vi "CreateS19Data.vi"(0 "SoftwareFilesPath [C:\\PRUEF]":string="C:\\PRUEF\\Programming\\001.001.001pre", 1 "Address [hex - 4bit]":u32=4198400 format="%08x", 2 "DataType":u16(ring) items=["ASCI", "FourByteCalData", "Hex"], 3 "Data [ASCII]":string="Empty", 4 "calData":u32 format="%.0x", 5 "Data":u8[](array[numeric]) format="%.0x", 6 "append?":bool) -> (19 "error out":errorcluster)   [LabVIEW 2012]
panel:
  out "spreadsheet string":string="S30B004010004FF003007047AB"
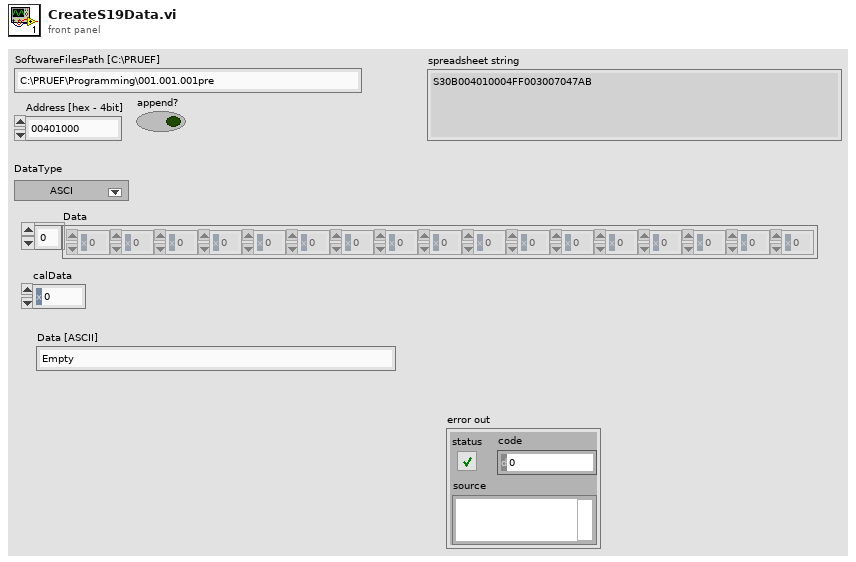
[diagram p1: front panel]
types:
  T1 = enum16{"open", "replace", "create", "open or create", "replace or create", "replace or create with confirmation"}
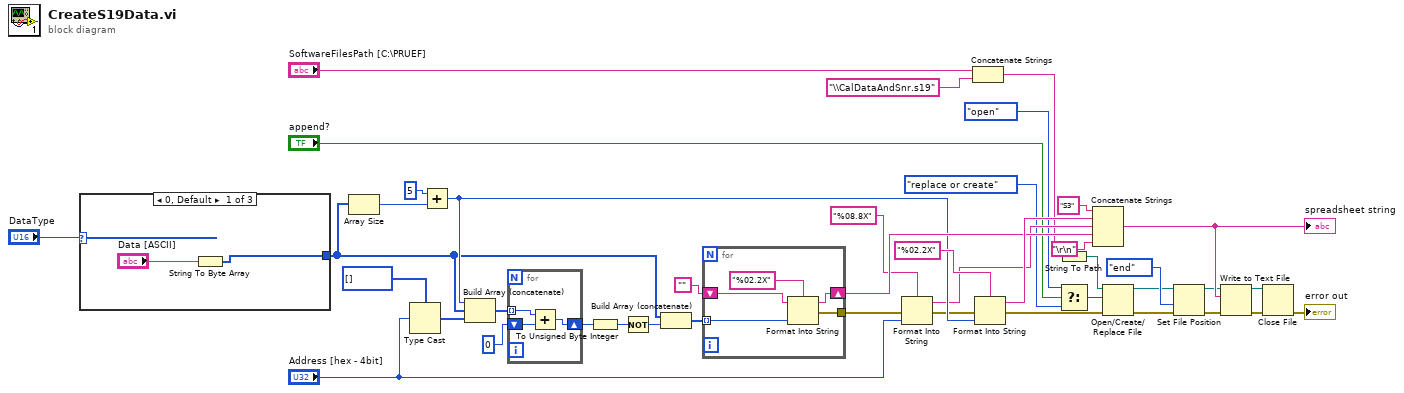
[diagram p0: block diagram]
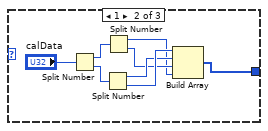
[diagram p2: hidden frame]
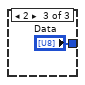
[diagram p3: hidden frame]
diagram:
  n1 = case shown="0, Default" "DataType" {
    tunnel: [w43 w45 "Data"] -> w12
    frame 0, Default {
      n2 = String To Byte Array(string="Data [ASCII]") -> (unsigned byte array=w43:u8[])
    }
    frame 1 {
      n3 = Split Number(x="calData") -> (hi(x)=w51:u16, lo(x)=w50:u16)
      n4 = Split Number(x=w50) -> (hi(x)=w48:u8, lo(x)=w49:u8)
      n5 = Split Number(x=w51) -> (hi(x)=w46:u8, lo(x)=w47:u8)
      n6 = Build Array(w49, w48, w47, w46) -> (w45:u8[])
    }
    frame 2 {
    }
  }
  n7 = Array Size(array=w12) -> (size(s)=w31:i32)
  n8 = Type Cast(type=u8[] [] ("array"), x="Address [hex - 4bit]") -> (*(type *) &x=w24:u8[])
  n9 = Add(x=5, y=w31) -> (x+y=w29:i32)
  n10 = Build Array (concatenate)(w29, w12, w24) -> (w39:i32[])
  n11 = for {
    shift-right: [w55] -> w40
    shift-left: 0 -> [w56]
    tunnel: w39 -> [w54] mode=indexing
    n12 = Add(x=w54, y=w56) -> (x+y=w55:i32)
  }
  n13 = To Unsigned Byte Integer(number=w40) -> (unsigned 8bit integer=w41:u8)
  n14 = Not(x=w41) -> (.not. x?=w38:u8)
  n15 = Build Array (concatenate)(w12, w38) -> (w34:u8[])
  n16 = for {
    tunnel: w34 -> [w61] mode=indexing
    shift-right: [w59] -> w32
    shift-left: "" -> [w58]
    tunnel: [w57] -> w23
    n17 = Format Into String(format string="%02.2X", initial string=w58, w61) -> (resulting string=w59:string, error out=w57:errorcluster)  [unwired: 1 in]
  }
  n18 = Format Into String(format string="%08.8X", error in=w23, "Address [hex - 4bit]") -> (resulting string=w27:string, error out=w22:errorcluster)  [unwired: 1 in]
  n19 = Concatenate Strings("SoftwareFilesPath [C:\\PRUEF]", "\\CalDataAndSnr.s19" ("string")) -> (w13:string)
  n20 = Format Into String(format string="%02.2X", error in=w22, w29) -> (resulting string=w35:string, error out=w21:errorcluster)  [unwired: 1 in]
  n21 = String To Path(string=w13) -> (path=w17:path)
  n22 = Select(t=T1."open", s="append?", f=T1."replace or create" ("operation (0:open)")) -> (s? t:f=w10:T1)
  n23 = Concatenate Strings("S3", w35, w27, w32, "\r\n") -> (w20:string)
  "spreadsheet string" <- w20
  n24 = Open/Create/Replace File(file path (use dialog)=w17, error in=w21, operation (0:open)=w10) -> (refnum out=w2:refnum<file>, error out=w3:errorcluster)  [unwired: 3 in, 1 out]
  n25 = Set File Position(refnum=w2, from (0:start)=enum16{"start", "end", "current"}."end", error in=w3) -> (refnum out=w1:refnum<file>, error out=w5:errorcluster)  [unwired: 1 in]
  n26 = Write to Text File(file (use dialog)=w1, text=w20, error in=w5) -> (refnum out=w19:refnum<file>, error out=w18:errorcluster)  [unwired: 1 in, 1 out]
  n27 = Close File(refnum=w19, error in=w18) -> (error out=→"error out":errorcluster)  [unwired: 1 out]
